vi "CombineQueueText.vi"(2 "Old List":string, 3 "Queue In":string) -> (1 "New List":string)   [LabVIEW 2016]
doc: "Combines the previous queue list with a new input"
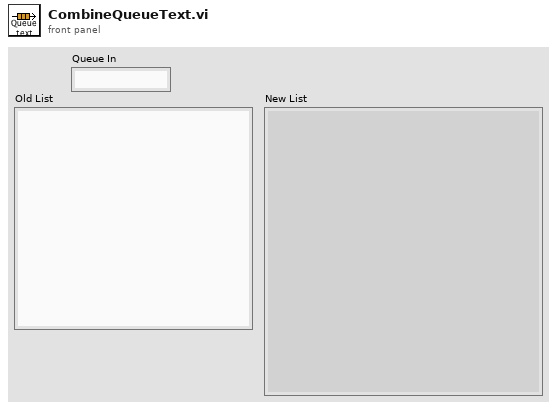
[diagram p1: front panel]
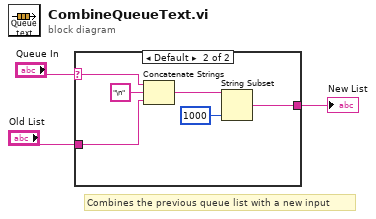
[diagram p0: block diagram]
diagram:
  # "Combines the previous queue list with a new input"
  n1 = case shown="Default" "Queue In" {
    selector: "Queue In" -> [_ w6]
    tunnel: [w4 w8] -> w3
    tunnel: "Old List" -> [w4 w5]
    frame "" {
    }
    frame Default {
      n2 = Concatenate Strings(w6, "\n" ("string"), w5) -> (w9:string)
      n3 = String Subset(string=w9, length (rest)=1000 ("length (rest)")) -> (substring=w8:string)  [unwired: 1 in]
    }
  }
  "New List" <- w3
